vi "Measurement UI.vi"() -> ()   [LabVIEW 2020, in "NIScopeAcquireWaveform.lvlib"]
uses:
  NIScopeAcquireWaveform.lvlib
panel:
  in  "Input Impedance":u32(ring) items=["1 mega ohm"=0, "50 ohms"=2]
  in  "Trigger Coupling":u32(ring) items=["AC"=0, "DC"=1, "HF Reject"=3, "LF Reject"=4, "AC Plus HF Reject"=1001]
  in  "Timeout":dbl
  in  "Trigger Slope":i32(ring) items=["Positive", "Negative"]
  in  "Trigger Level":dbl
  in  "Trigger Source":string(combo)
  in  "Minimum Record Length":i32
  in  "Minimum Sample Rate":dbl
  in  "Vertical Coupling":i32(ring) items=["AC", "DC", "Ground"]
  in  "Pin Names":string[](array[combo])
  in  "Vertical Range":dbl
  out "Waveform3":dbl[](array[numeric])
  out "Waveform2":dbl[](array[numeric])
  out "Waveform1":dbl[](array[numeric])
  out "Waveform0":dbl[](array[numeric])
  out "Waveform Graph":dbl[][](graph)
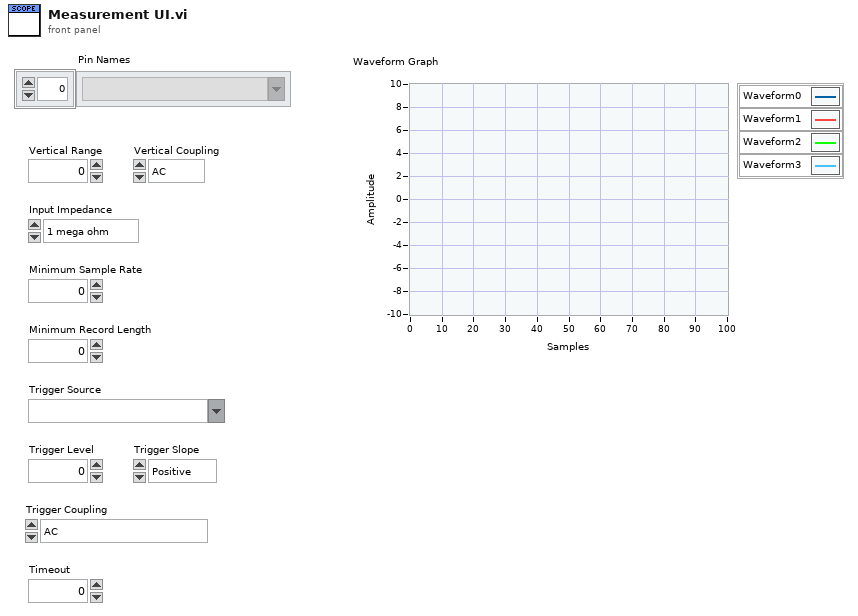
[diagram p1: front panel]
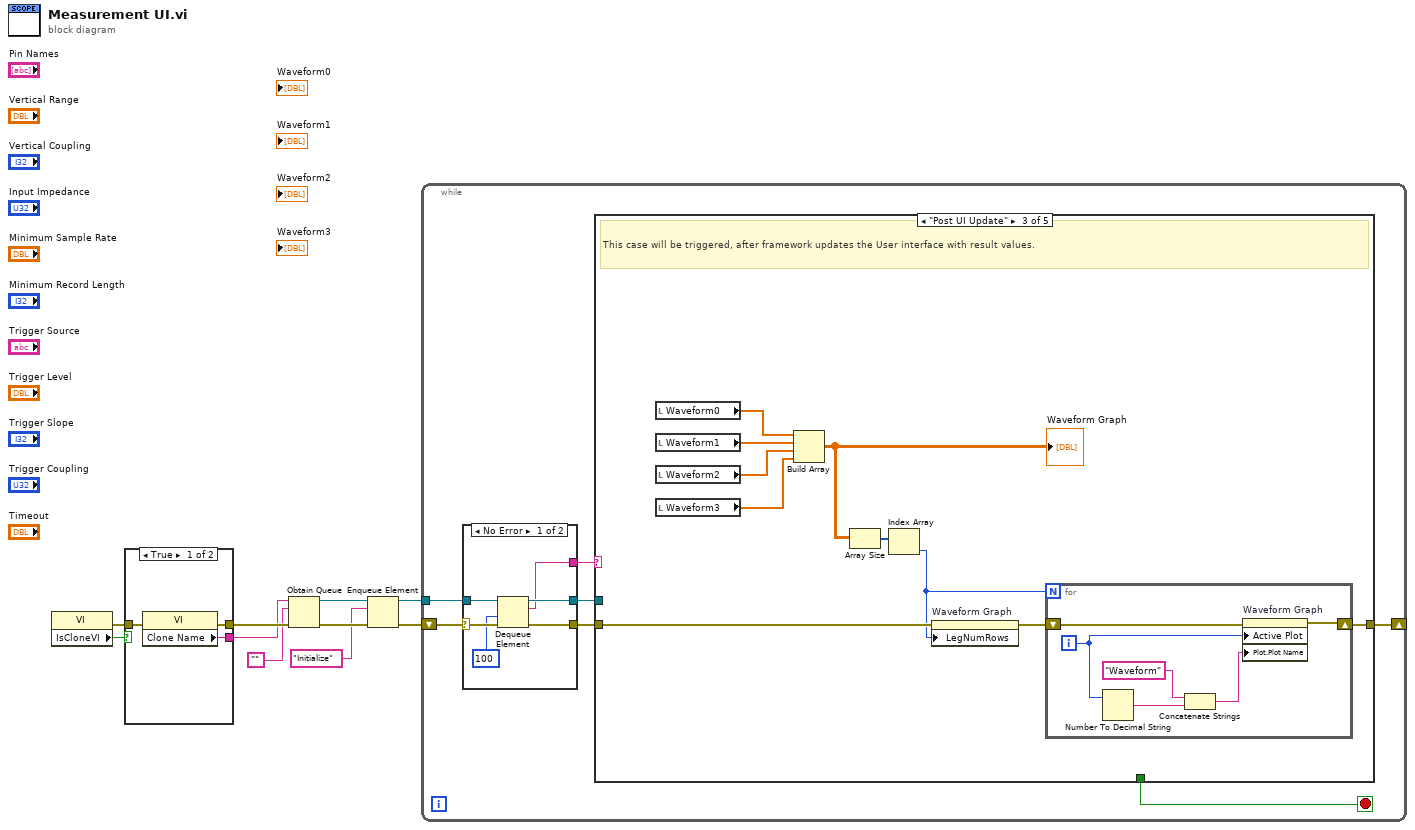
[diagram p0: block diagram]
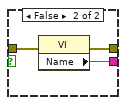
[diagram p2: hidden frame]
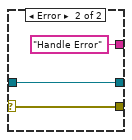
[diagram p3: hidden frame]
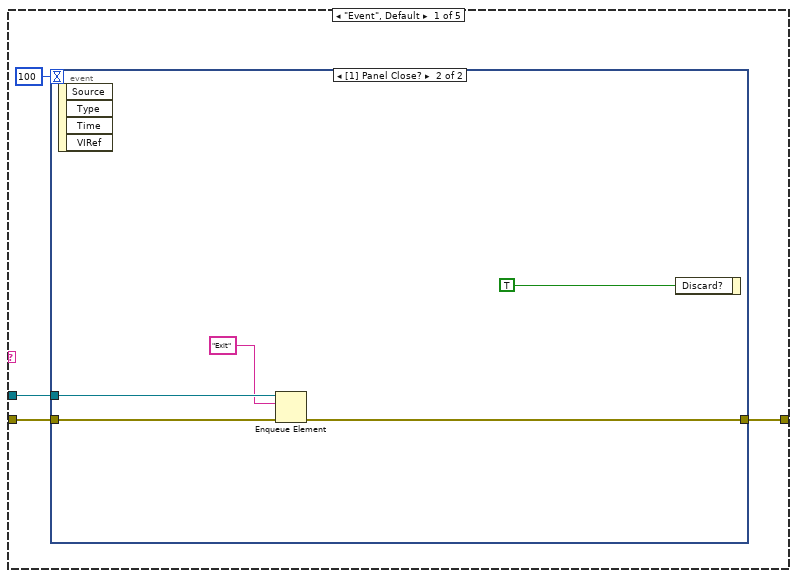
[diagram p4: hidden frame]
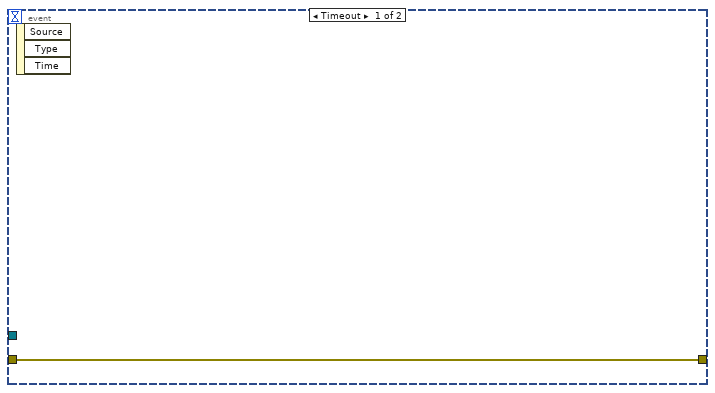
[diagram p5: hidden frame]
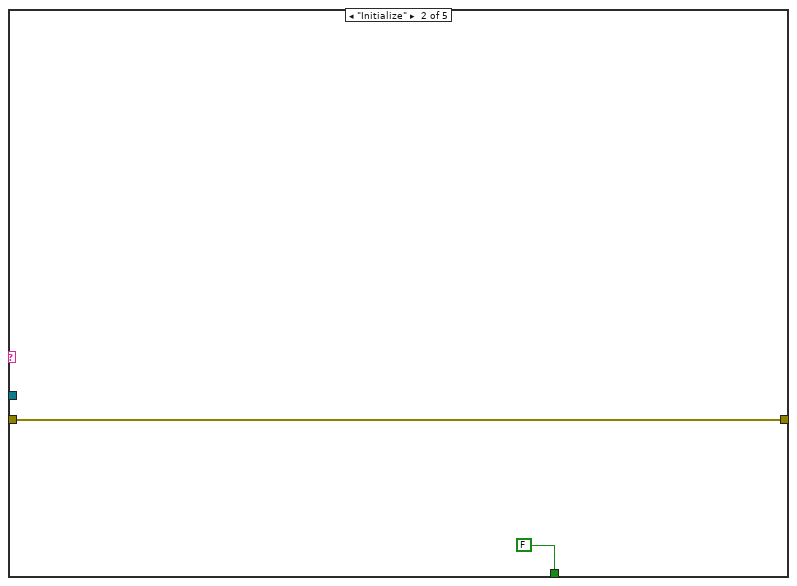
[diagram p6: hidden frame]
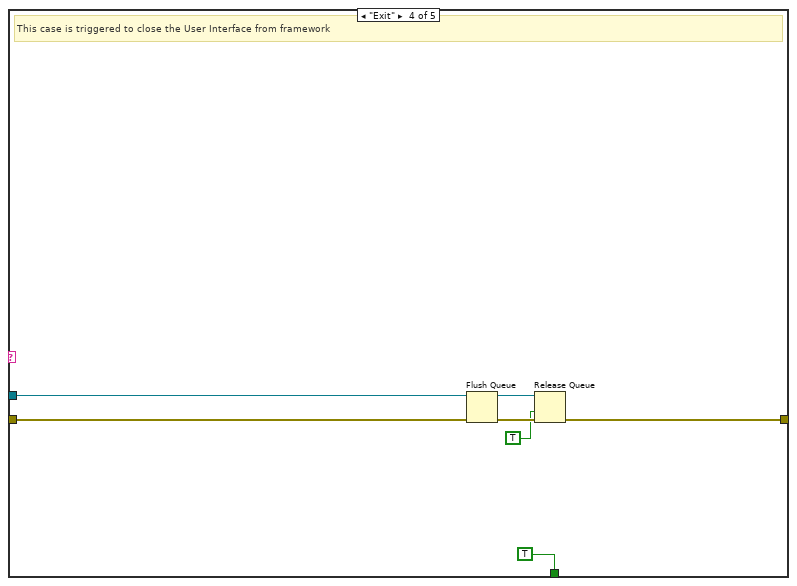
[diagram p7: hidden frame]
diagram:
  n1 = property class="VI"() -> (error out=w1:errorcluster, "IsCloneVI"=w2:bool)  [unwired: 2 in, 1 out]
  n2 = case shown="True" w2 {
    tunnel: [w13 w16] -> w10
    tunnel: [w12 w15] -> w9
    tunnel: w1 -> [w11 w14]
    frame True {
      n3 = property class="VI"(error in=w11) -> (error out=w13:errorcluster, "Clone Name"=w12:string)  [unwired: 1 in, 1 out]
    }
    frame False {
      n4 = property class="VI"(error in=w14) -> (error out=w16:errorcluster, "Name"=w15:string)  [unwired: 1 in, 1 out]
    }
  }
  n5 = Obtain Queue(name (unnamed)=w9, element data type="", error in (no error)=w10) -> (queue out=w6:refnum<queue>, error out=w8:errorcluster)  [unwired: 2 in, 1 out]
  n6 = Enqueue Element(queue=w6, element="Initialize", error in (no error)=w8) -> (queue out=w5:refnum<queue>, error out=w7:errorcluster)  [unwired: 1 in, 1 out]
  n7 = while {
    shift-right: [w18] -> _
    shift-left: w7 -> [w23]
    tunnel: w5 -> [w21]
    stop <- w17 stop-if-true
    n8 = case shown="No Error" w23 {
      selector: w23 -> [w29 w32]
      tunnel: [w28 w32] -> w22
      tunnel: w21 -> [w27 w31]
      tunnel: [w26 w31] -> w20
      tunnel: [w25 "Handle Error"] -> w19
      frame No Error {
        n9 = Dequeue Element(queue=w27, timeout in ms (-1)=100, error in (no error)=w29) -> (queue out=w26:refnum<queue>, element=w25:string, error out=w28:errorcluster)  [unwired: 1 out]
      }
      frame Error {
      }
    }
    n10 = case shown="\"Post UI Update\"" w19 {
      tunnel: w22 -> [w35 w44 w50 w67 w68]
      tunnel: w20 -> [w33 _ _ w65 _]
      tunnel: [w36 w44 w48 w62 w68] -> w18
      tunnel: [_ FALSE _ TRUE _] -> w17
      frame "Event", Default {
        n11 = event shown="[1] Panel Close?" {
          selector: _ -> [_ _]
          dyn-events: _ -> [_ _]
          timeout: 100 -> [_ _]
          tunnel: [w37 w40] -> w36
          tunnel: w35 -> [w37 w41]
          tunnel: w33 -> [_ w39]
          event Timeout {
            n12 = event-data() -> ()  [unwired: 1 in, 3 out]
          }
          event Panel Close? {
            n13 = event-data() -> ()  [unwired: 1 in, 4 out]
            n14 = Enqueue Element(queue=w39, element="Exit", error in (no error)=w41) -> (error out=w40:errorcluster)  [unwired: 1 in, 2 out]
            n15 = event-data("Discard?"=TRUE) -> ()  [unwired: 1 in, 1 out]
          }
        }
      }
      frame "Initialize" {
      }
      frame "Post UI Update" {
        # "This case will be triggered, after framework updates the User interface with result values."
        n16 = local read "Waveform0"() -> (w54:dbl[])
        n17 = local read "Waveform1"() -> (w53:dbl[])
        n18 = local read "Waveform2"() -> (w52:dbl[])
        n19 = local read "Waveform3"() -> (w51:dbl[])
        n20 = Build Array(w54, w53, w52, w51) -> (w47:dbl[][])
        "Waveform Graph" <- w47
        n21 = Array Size(array=w47) -> (size(s)=w46:i32[])
        n22 = Index Array(array=w46) -> (element=w45:i32)  [unwired: 1 in]
        n23 = property on="Waveform Graph" class="WFGraph (strict)"(error in=w50, "LegNumRows"=w45) -> (error out=w49:errorcluster)  [unwired: 1 in, 1 out]
        n24 = for {
          N: w45 -> [_]
          shift-right: [w59] -> w48
          shift-left: w49 -> [w60]
          i -> [w58]
          n25 = Number To Decimal String(number=w58) -> (decimal integer string=w56:string)  [unwired: 1 in]
          n26 = Concatenate Strings("Waveform", w56) -> (w55:string)
          n27 = property on="Waveform Graph" class="WFGraph (strict)"(error in=w60, "Active Plot"=w58, "Plot.Plot Name"=w55) -> (error out=w59:errorcluster)  [unwired: 1 in, 1 out]
        }
      }
      frame "Exit" {
        # "This case is triggered to close the User Interface from framework"
        n28 = Flush Queue(queue=w65, error in (no error)=w67) -> (queue out=w64:refnum<queue>, error out=w63:errorcluster)  [unwired: 1 out]
        n29 = Release Queue(queue=w64, force destroy? (F)=TRUE, error in (no error)=w63) -> (error out=w62:errorcluster)  [unwired: 2 out]
      }
      frame "Handle Error" {
      }
    }
  }
